vi "Update_Grid_Res_Drift_Correction_SubVI.vi"(9 "Drift Correction Settings":T2, 10 "Boolean":bool, 11 "Experiment 6":T1) -> (3 "Experiment 5":T1)   [LabVIEW 2014]
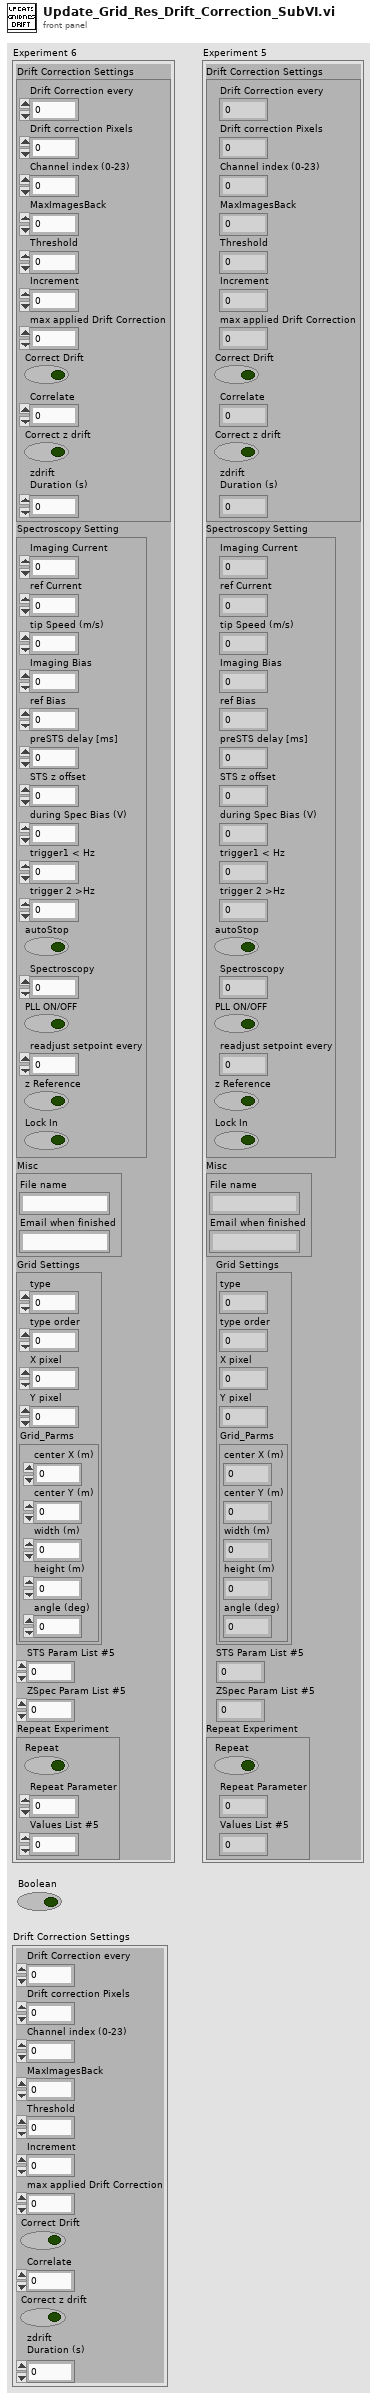
[diagram p1: front panel]
types:
  T1 = cluster{"Drift Correction Settings":cluster{"Drift Correction every":i32, "Drift correction Pixels":i32, "Channel index (0-23)":u8, "MaxImagesBack":i32, "Threshold":i32, "Increment":i32, "max applied Drift Correction":i32, "Correct Drift":bool, "Correlate":u16, "Correct z drift":bool, "zdrift \nDuration (s)":dbl}, "Spectroscopy Setting":cluster{"Imaging Current":dbl, "ref Current":dbl, "tip Speed (m/s)":sgl, "Imaging Bias":dbl, "ref Bias":dbl, "preSTS delay [ms]":u32, "STS z offset":dbl, "during Spec Bias (V)":sgl, "trigger1 < Hz":sgl, "trigger 2 >Hz":sgl, "autoStop":bool, "Spectroscopy":u16, "PLL ON/OFF":bool, "readjust setpoint every ":i32, "z Reference":bool, "Lock In":bool}, "Misc":cluster{"File name":string, "Email when finished":string}, "Grid Settings":cluster{"type":u16, "type order":u16, "X pixel":i32, "Y pixel":i32, "Grid_Parms":cluster{"center X (m)":sgl, "center Y (m)":sgl, "width (m)":sgl, "height (m)":sgl, "angle (deg)":sgl}}, "STS Param List #5 ":u16, "ZSpec Param List #5  ":u16, "Repeat Experiment":cluster{"Repeat":bool, "Repeat Parameter":u16, "Values List #5":i32}}
  T2 = cluster{"Drift Correction every":i32, "Drift correction Pixels":i32, "Channel index (0-23)":u8, "MaxImagesBack":i32, "Threshold":i32, "Increment":i32, "max applied Drift Correction":i32, "Correct Drift":bool, "Correlate":u16, "Correct z drift":bool, "zdrift \nDuration (s)":dbl}
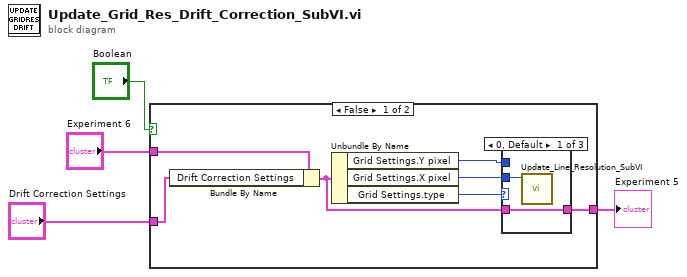
[diagram p0: block diagram]
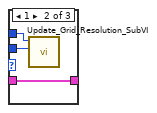
[diagram p2: hidden frame]
diagram:
  n1 = case shown="False" "Boolean" {
    tunnel: [w11 w18] -> w4
    tunnel: "Experiment 6" -> [w7 w18]
    tunnel: "Drift Correction Settings" -> [w6 _]
    frame False {
      n2 = Bundle By Name(cluster=w7, "Drift Correction Settings"=w6) -> (w8:T1)
      n3 = Unbundle By Name(w8) -> ("Grid Settings.Y pixel"=w9:i32, "Grid Settings.X pixel"=w10:i32, "Grid Settings.type"=w5:u16)
      n4 = case shown="0, Default" w5 {
        tunnel: w8 -> [w13 w14 w17]
        tunnel: [w13 w14 w17] -> w11
        tunnel: w10 -> [w12 w16 _]
        tunnel: w9 -> [_ w15 _]
        frame 0, Default {
          n5 = call "Update_Line_Resolution_SubVI.vi"("X pixel"=w12) -> ()  [unwired: 11 in]
        }
        frame 1 {
          n6 = call "Update_Grid_Resolution_SubVI.vi"("X pixel"=w16, "Y pixel"=w15) -> ()  [unwired: 10 in]
        }
        frame 2 {
        }
      }
    }
    frame True {
    }
  }
  "Experiment 5" <- w4
